vi "LVClass_SlopesPostProcessList GetParameter_Substractor.vi"(0 "SlopesPostProcessorList in":refnum<class "SlopesPostProcessorList.lvclass">, 5 "Position":u32, 7 "HasoSlopes.lvclass":refnum<class "HasoSlopes.lvclass">, 11 "error in (no error)":errorcluster) -> (4 "SlopesPostProcessorList out":refnum<class "SlopesPostProcessorList.lvclass">, 8 "hasoslopes":refnum<class "HasoSlopes.lvclass">, 10 "Comment":string, 15 "error out":errorcluster)   [LabVIEW 2020, in "SlopesPostProcessorList.lvclass"]
doc: "Get parameters of the Substractor processor.\n\n--------------------------------------------------------------------------------\n\n<B>SlopesPostProcessorListIn </B> : SlopesPostProcessorList object.\n<B>SlopesPostProcessorListOut </B> : SlopesPostProcessorList object.\n<B>position </B> : Position of the processor in the SlopesPostProcessorList.\n<B>comment </B> : Comments.\n<B>hasoslopes </B> : HasoSlopes to set in the processor.\n<B>ErrorIn </B> : Error\n<B>ErrorOut </B> : Error\n\n--------------------------------------------------------------------------------"
uses:
  SlopesPostProcessorList.lvclass
  HasoSlopes/HasoSlopes.lvclass
  SlopesPostProcessorList.lvclass/SlopesPostProcessorList.ctl
  HasoSlopes/LVClass_HasoSlopes Read HasoSlopes _ property.vi
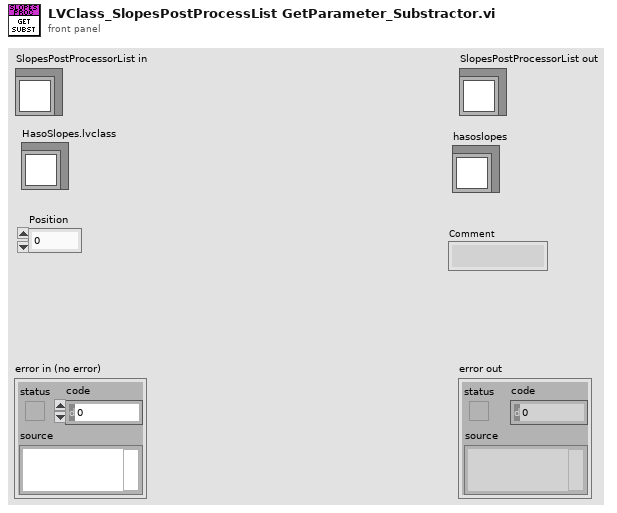
[diagram p1: front panel]
types:
  T1 = typedef "ClassID.ctl" = i64
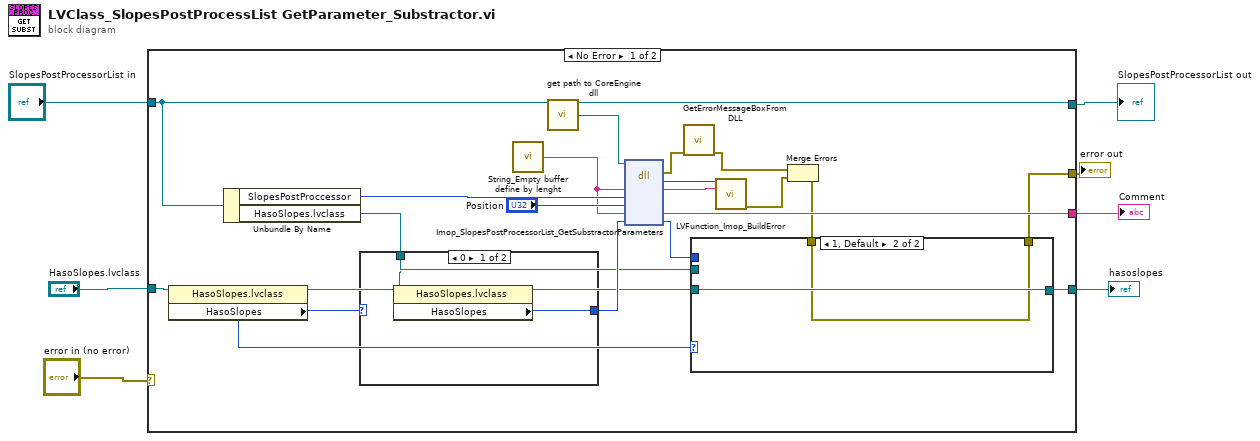
[diagram p0: block diagram]
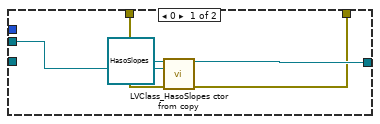
[diagram p2: hidden frame]
diagram:
  n1 = case shown="No Error" "error in (no error)" {
    selector: "error in (no error)" -> [_ w39]
    tunnel: "SlopesPostProcessorList in" -> [w23 w40]
    tunnel: [w23 w40] -> w5
    tunnel: [w8 w39] -> w4
    tunnel: "HasoSlopes.lvclass" -> [w21 w38]
    tunnel: [w11 w38] -> w2
    tunnel: [w16 _] -> w1
    frame No Error {
      n2 = property class="HasoSlopes.lvclass"(reference=w21) -> (reference out=w10:refnum<class "HasoSlopes.lvclass">, "HasoSlopes"=w14:T1)  [unwired: 1 in, 1 out]
      n3 = Unbundle By Name(w23) -> ("SlopesPostProccessor"=w22:T1, "HasoSlopes.lvclass"=w12:refnum<class "HasoSlopes.lvclass">)
      n4 = case shown="0" w14 {
        selector: w14 -> [_ w37]
        tunnel: w12 -> [w36 _]
        tunnel: [w35 w37] -> w15
        frame 0 {
          n5 = property class="HasoSlopes.lvclass"(reference=w36) -> ("HasoSlopes"=w35:T1)  [unwired: 1 in, 2 out]
        }
        frame 1, Default {
        }
      }
      n6 = call "String_Empty buffer define by lenght.vi"() -> ("Empty buffer"=w17:string)  [unwired: 1 in]
      n7 = call "get path to CoreEngine dll.vi"() -> ("path to wavekit library"=w25:path)  [unwired: 14 in, 1 out]
      n8 = dll-call lib="D:/soft/HASO_v3/SVN_trunk/ImOpCoreEngine4_LV2011/DLLs/c_interface_vc100.dll" fn="Imop_SlopesPostProcessorList_GetSubstractorParameters"(path in=w25, "message"=w17, "objet"=w22, "Position"="Position", "Comment"=w17, "hasoslopes"=w15) -> (error out=w24:errorcluster, "return type"=w26:i32, "message"=w27:string, "Comment"=w16:string, "hasoslopes"=w13:i64)  [unwired: 4 in, 1 out]
      n9 = call "GetErrorMessageBoxFromDLL.vi"("error IN"=w24) -> ("error OUT"=w19:errorcluster)  [unwired: 10 in]
      n10 = call "LVFunction_Imop_BuildError.vi"("code"=w26, "String to Prepend to source (\"\")"=w27) -> ("error out"=w18:errorcluster)  [unwired: 13 in]
      n11 = Merge Errors(w19, w18) -> (w9:errorcluster)
      n12 = case shown="1, Default" w14 {
        tunnel: w13 -> [_ _]
        tunnel: w12 -> [w31 _]
        tunnel: [w29 w34] -> w11
        tunnel: w10 -> [_ w34]
        tunnel: w9 -> [w30 w33]
        tunnel: [w28 w33] -> w8
        frame 0 {
          n13 = call "LVClass_HasoSlopes ctor from copy.vi"("HasoSlopes (const)"=refnum<class "HasoSlopes.lvclass"> refnum ("HasoSlopes in"), "HasoSlopes ToCopy"=w31, "error in (no error)"=w30) -> ("HasoSlopes (new)"=w29:refnum<class "HasoSlopes.lvclass">, "error out"=w28:errorcluster)  [unwired: 10 in, 1 out]
        }
        frame 1, Default {
        }
      }
    }
    frame Error {
    }
  }
  "error out" <- w4
  "SlopesPostProcessorList out" <- w5
  "hasoslopes" <- w2
  "Comment" <- w1
